vi "get_centroid.vi"(8 "error in (no error)":errorcluster, 11 "TrajectoryDL110420DoubleCircle in":refnum<class "TrajectoryDL110420DoubleCircle.lvclass">) -> (0 "error out":errorcluster, 2 "centroid":refnum<class "SpaceVector.lvclass">, 3 "TrajectoryDL110420DoubleCircle out":refnum<class "TrajectoryDL110420DoubleCircle.lvclass">)   [LabVIEW 2010, in "TrajectoryDL110420DoubleCircle.lvclass"]
uses:
  TrajectoryDL110420DoubleCircle.lvclass
  common/classes/SpaceVector/SpaceVector/SpaceVector.lvclass
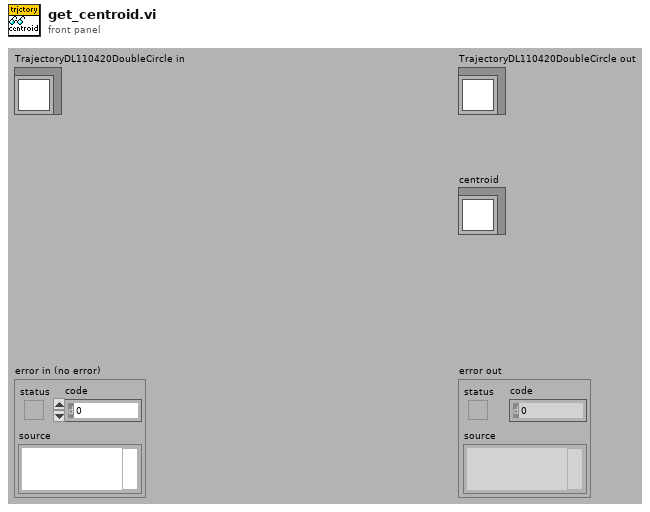
[diagram p1: front panel]
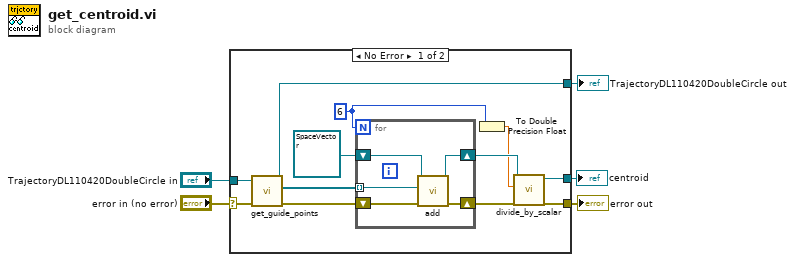
[diagram p0: block diagram]
diagram:
  n1 = case shown="No Error" "error in (no error)" {
    selector: "error in (no error)" -> [w7 w24]
    tunnel: [w16 w24] -> w4
    tunnel: [w8 w23] -> w2
    tunnel: "TrajectoryDL110420DoubleCircle in" -> [w9 w23]
    tunnel: [w17 _] -> w1
    frame No Error {
      w12 = 6
      n2 = call-dynamic "get_guide_points.vi"("error in (no error)"=w7, "TrajectoryDL110420DoubleCircle in"=w9) -> ("error out"=w6:errorcluster, "guide points"=w10:refnum<class "SpaceVector.lvclass">[], "TrajectoryDL110420DoubleCircle out"=w8:refnum<class "TrajectoryDL110420DoubleCircle.lvclass">)  [unwired: 7 in]
      n3 = for {
        N: w12 -> [_]
        shift-right: [w18] -> w14
        shift-left: w6 -> [w22]
        tunnel: w10 -> [w20] mode=indexing
        shift-right: [w19] -> w13
        shift-left: refnum<class "SpaceVector.lvclass"> refnum ("SpaceVector.lvclass") -> [w21]
        n4 = call "add.vi"("error in (no error)"=w22, "vector to be added"=w20, "SpaceVector in"=w21) -> ("error out"=w18:errorcluster, "SpaceVector out"=w19:refnum<class "SpaceVector.lvclass">)  [unwired: 7 in]
      }
      n5 = To Double Precision Float(number=w12) -> (double precision float=w11:dbl)
      n6 = call "divide_by_scalar.vi"("error in (no error)"=w14, "divisor"=w11, "SpaceVector in"=w13) -> ("error out"=w16:errorcluster, "SpaceVector out"=w17:refnum<class "SpaceVector.lvclass">)  [unwired: 7 in]
    }
    frame Error {
    }
  }
  "error out" <- w4
  "TrajectoryDL110420DoubleCircle out" <- w2
  "centroid" <- w1
